vi "GEN_Error Info.vi"(8 "error in":errorcluster caption="错误输入（无错误）", 10 "Event name":string, 11 "Thread name":string) -> (0 "error out":errorcluster caption="错误输出", 2 "Error Report":string)   [LabVIEW 2016]
uses:
  <vilib>/Utility/error.llb/DialogType.ctl
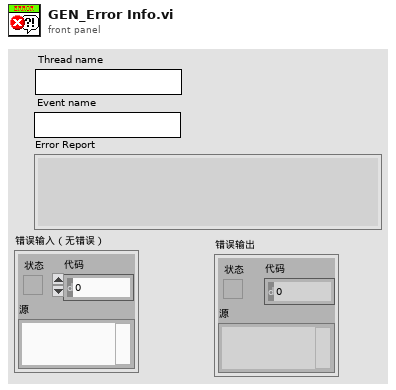
[diagram p1: front panel]
types:
  T1 = typedef "DialogType.ctl" = u16
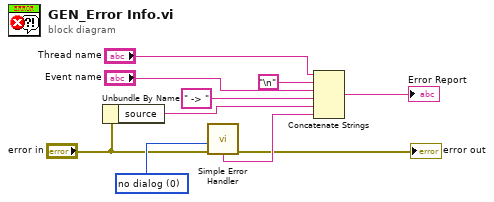
[diagram p0: block diagram]
diagram:
  w10 = T1 0 items=["no dialog", "OK message", "continue or stop message", "OK message + warnings", "continue/stop + warnings"] ("type of dialog (OK msg:1)")
  n1 = Unbundle By Name("error in") -> ("source"=w4:string)
  n2 = call <vilib>:"Simple Error Handler.vi"("type of dialog (OK msg:1)"=w10, "error in (no error)"="error in") -> ("error out"=→"error out":errorcluster, "message"=w8:string)  [unwired: 3 in, 3 out]
  n3 = Concatenate Strings("Thread name", "\n", "Event name", " -> " ("字符串"), w4, w8) -> (→"Error Report":string)
